vi "VI_Tree.vi"   [LabVIEW 2018, in "Seimens.lvclass"]
uses:
  Seimens.lvclass
  Read/SeimensS7Net_ReadBool.vi
  Read/SeimensS7Net_ReadByte.vi
  Read/SeimensS7Net_ReadByte[].vi
  Read/SeimensS7Net_ReadDouble.vi
  Read/SeimensS7Net_ReadDouble[].vi
  Read/SeimensS7Net_ReadFloat.vi
  Read/SeimensS7Net_ReadInt32.vi
  Read/SeimensS7Net_ReadInt32[].vi
  Read/SeimensS7Net_ReadInt16.vi
  Read/SeimensS7Net_ReadInt16[].vi
  Read/SeimensS7Net_ReadString.vi
  Read/SeimensS7Net_ReadString[].vi
  Read/SeimensS7Net_ReadUInt16.vi
  Read/SeimensS7Net_ReadUInt16[].vi
  Read/SeimensS7Net_ReadInt64.vi
  Read/SeimensS7Net_ReadInt64[].vi
  Read/SeimensS7Net_ReadUInt32.vi
  Read/SeimensS7Net_ReadUInt32[].vi
  Read/SeimensS7Net_ReadUInt64.vi
  Read/SeimensS7Net_ReadUInt64[].vi
  Write/SeimensS7Net_WriteBool.vi
  Write/SeimensS7Net_WriteByte.vi
  Write/SeimensS7Net_WriteInt16.vi
  Write/SeimensS7Net_WriteInt16[].vi
  Write/SeimensS7Net_WriteInt32.vi
  Write/SeimensS7Net_WriteInt32[].vi
  Write/SeimensS7Net_WriteInt64.vi
  Write/SeimensS7Net_WriteInt64[].vi
  Write/SeimensS7Net_WriteFloat.vi
  Write/SeimensS7Net_WriteFloat[].vi
  Write/SeimensS7Net_WriteDouble.vi
  Write/SeimensS7Net_WriteDouble[].vi
  Write/SeimensS7Net_WriteUInt16.vi
  Write/SeimensS7Net_WriteUInt16[].vi
  Write/SeimensS7Net_WriteUInt32.vi
  Write/SeimensS7Net_WriteUInt32[].vi
  Write/SeimensS7Net_WriteUInt64.vi
  Write/SeimensS7Net_WriteUInt64[].vi
  Write/SeimensS7Net_WriteString.vi
  Write/SeimensS7Net_WriteString[].vi
  Write/SeimensS7Net_WriteByte[].vi
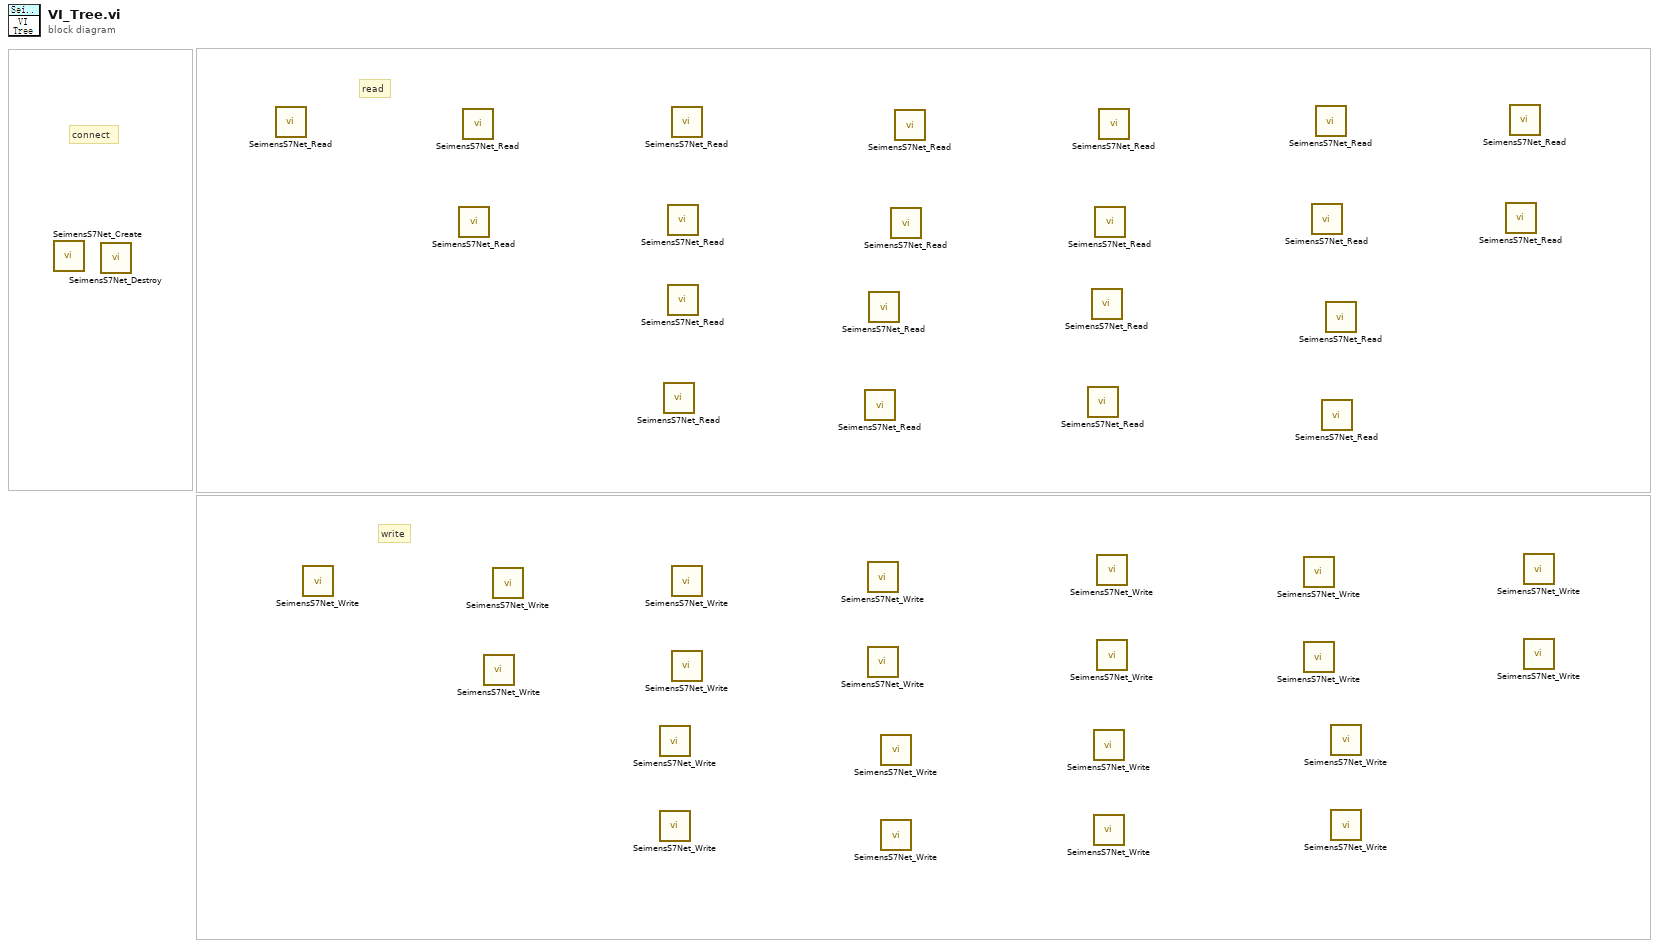
[diagram p0: block diagram]
diagram:
  # "write"
  # "read"
  # "connect"
  n1 = call "SeimensS7Net_Create.vi"() -> ()  [unwired: 10 in, 2 out]
  n2 = call "SeimensS7Net_Destroy.vi"() -> ()  [unwired: 11 in, 1 out]
  n3 = call-poly "SeimensS7Net_Read.vi"() -> ()  [unwired: 9 in, 3 out]
  n4 = call-poly "SeimensS7Net_Write.vi"() -> ()  [unwired: 10 in, 2 out]
  n5 = call-poly "SeimensS7Net_Read.vi"() -> ()  [unwired: 9 in, 3 out]
  n6 = call-poly "SeimensS7Net_Read.vi"() -> ()  [unwired: 9 in, 3 out]
  n7 = call-poly "SeimensS7Net_Write.vi"() -> ()  [unwired: 9 in, 3 out]
  n8 = call-poly "SeimensS7Net_Write.vi"() -> ()  [unwired: 10 in, 2 out]
  n9 = call-poly "SeimensS7Net_Write.vi"() -> ()  [unwired: 10 in, 2 out]
  n10 = call-poly "SeimensS7Net_Write.vi"() -> ()  [unwired: 9 in, 3 out]
  n11 = call-poly "SeimensS7Net_Read.vi"() -> ()  [unwired: 9 in, 3 out]
  n12 = call-poly "SeimensS7Net_Read.vi"() -> ()  [unwired: 9 in, 3 out]
  n13 = call-poly "SeimensS7Net_Read.vi"() -> ()  [unwired: 9 in, 3 out]
  n14 = call-poly "SeimensS7Net_Read.vi"() -> ()  [unwired: 9 in, 3 out]
  n15 = call-poly "SeimensS7Net_Write.vi"() -> ()  [unwired: 10 in, 2 out]
  n16 = call-poly "SeimensS7Net_Write.vi"() -> ()  [unwired: 9 in, 3 out]
  n17 = call-poly "SeimensS7Net_Read.vi"() -> ()  [unwired: 9 in, 3 out]
  n18 = call-poly "SeimensS7Net_Write.vi"() -> ()  [unwired: 10 in, 2 out]
  n19 = call-poly "SeimensS7Net_Write.vi"() -> ()  [unwired: 9 in, 3 out]
  n20 = call-poly "SeimensS7Net_Read.vi"() -> ()  [unwired: 9 in, 3 out]
  n21 = call-poly "SeimensS7Net_Write.vi"() -> ()  [unwired: 10 in, 2 out]
  n22 = call-poly "SeimensS7Net_Write.vi"() -> ()  [unwired: 9 in, 3 out]
  n23 = call-poly "SeimensS7Net_Read.vi"() -> ()  [unwired: 9 in, 3 out]
  n24 = call-poly "SeimensS7Net_Read.vi"() -> ()  [unwired: 9 in, 3 out]
  n25 = call-poly "SeimensS7Net_Read.vi"() -> ()  [unwired: 9 in, 3 out]
  n26 = call-poly "SeimensS7Net_Read.vi"() -> ()  [unwired: 9 in, 3 out]
  n27 = call-poly "SeimensS7Net_Write.vi"() -> ()  [unwired: 10 in, 2 out]
  n28 = call-poly "SeimensS7Net_Write.vi"() -> ()  [unwired: 9 in, 3 out]
  n29 = call-poly "SeimensS7Net_Read.vi"() -> ()  [unwired: 9 in, 3 out]
  n30 = call-poly "SeimensS7Net_Write.vi"() -> ()  [unwired: 10 in, 2 out]
  n31 = call-poly "SeimensS7Net_Write.vi"() -> ()  [unwired: 9 in, 3 out]
  n32 = call-poly "SeimensS7Net_Read.vi"() -> ()  [unwired: 9 in, 3 out]
  n33 = call-poly "SeimensS7Net_Write.vi"() -> ()  [unwired: 10 in, 2 out]
  n34 = call-poly "SeimensS7Net_Write.vi"() -> ()  [unwired: 9 in, 3 out]
  n35 = call-poly "SeimensS7Net_Read.vi"() -> ()  [unwired: 9 in, 3 out]
  n36 = call-poly "SeimensS7Net_Read.vi"() -> ()  [unwired: 9 in, 3 out]
  n37 = call-poly "SeimensS7Net_Read.vi"() -> ()  [unwired: 9 in, 3 out]
  n38 = call-poly "SeimensS7Net_Read.vi"() -> ()  [unwired: 9 in, 3 out]
  n39 = call-poly "SeimensS7Net_Write.vi"() -> ()  [unwired: 10 in, 2 out]
  n40 = call-poly "SeimensS7Net_Write.vi"() -> ()  [unwired: 10 in, 2 out]
  n41 = call-poly "SeimensS7Net_Read.vi"() -> ()  [unwired: 9 in, 3 out]
  n42 = call-poly "SeimensS7Net_Read.vi"() -> ()  [unwired: 9 in, 3 out]
  n43 = call-poly "SeimensS7Net_Write.vi"() -> ()  [unwired: 10 in, 2 out]
  n44 = call-poly "SeimensS7Net_Write.vi"() -> ()  [unwired: 9 in, 3 out]
